vi "MOCKBEAR_Setter.vi"(8 "error in (no error)":errorcluster, 10 "Mockbear input controls":T1, 11 "MOCKBEAR in":refnum<class "MOCKBEAR.lvclass">) -> (0 "error out":errorcluster, 3 "MOCKBEAR out":refnum<class "MOCKBEAR.lvclass">)   [LabVIEW 2021, in "MOCKBEAR.lvclass"]
uses:
  MOCKBEAR.lvclass
  MOCKBEAR.lvclass/MOCKBEAR.ctl
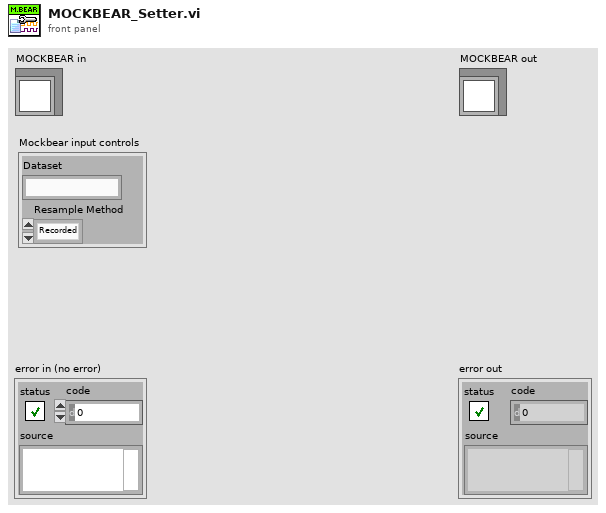
[diagram p1: front panel]
types:
  T1 = cluster{"Dataset":string, "Resample Method":enum16{"Recorded", "Auto Resample", "Custom Resample"}}
  T2 = enum16{"Recorded", "Auto Resample", "Custom Resample"}
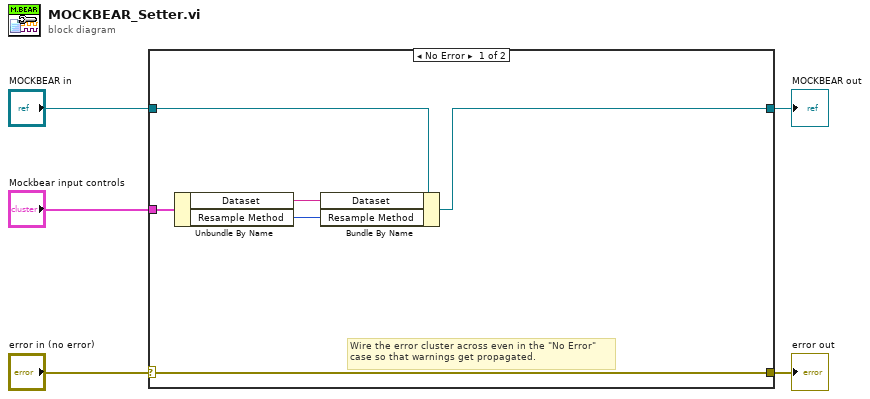
[diagram p0: block diagram]
diagram:
  n1 = case shown="No Error" "error in (no error)" {
    selector: "error in (no error)" -> [w11 w13]
    tunnel: [w11 w13] -> w4
    tunnel: [w6 w12] -> w2
    tunnel: "MOCKBEAR in" -> [w9 w12]
    tunnel: "Mockbear input controls" -> [w10 _]
    frame No Error {
      # "Wire the error cluster across even in the \"No Error\"\ncase so that warnings get propagated."
      n2 = Unbundle By Name(w10) -> ("Dataset"=w7:string, "Resample Method"=w8:T2)
      n3 = Bundle By Name(cluster=w9, "Dataset"=w7, "Resample Method"=w8) -> (w6:refnum<class "MOCKBEAR.lvclass">)
    }
    frame Error {
    }
  }
  "error out" <- w4
  "MOCKBEAR out" <- w2
